vi "PiezoDAQStop.vi"(9 "error in (no error)":errorcluster) -> (0 "Last Value":dbl, 6 "error out":errorcluster)   [LabVIEW 2009]
uses:
  PiezoGlobal.vi
  Program Files/National Instruments/LabVIEW 2009/resource/objmgr/daqmx.rc
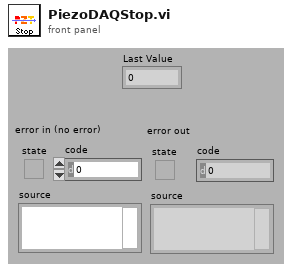
[diagram p1: front panel]
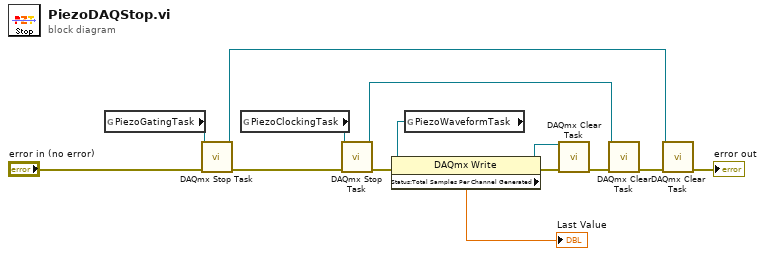
[diagram p0: block diagram]
diagram:
  n1 = global read "PiezoGlobal.vi" "PiezoGatingTask"() -> (w6:refnum<k21>)
  n2 = call <vilib>:"DAQmx Stop Task.vi"("task/channels in"=w6, "error in"="error in (no error)") -> ("task out"=w1:refnum<k21>, "error out"=w4:errorcluster)  [unwired: 12 in]
  n3 = global read "PiezoGlobal.vi" "PiezoClockingTask"() -> (w14:refnum<k21>)
  n4 = call <vilib>:"DAQmx Stop Task.vi"("task/channels in"=w14, "error in"=w4) -> ("task out"=w13:refnum<k21>, "error out"=w11:errorcluster)  [unwired: 12 in]
  n5 = global read "PiezoGlobal.vi" "PiezoWaveformTask"() -> (w10:refnum<k21>)
  n6 = property class="DAQmx Write"(reference=w10, error in=w11) -> (reference out=w9:refnum<k21>, error out=w8:errorcluster, "Status:Total Samples Per Channel Generated"=→"Last Value":dbl)
  n7 = call <vilib>:"DAQmx Clear Task.vi"("task in"=w9, "error in"=w8) -> ("error out"=w12:errorcluster)  [unwired: 13 in]
  n8 = call <vilib>:"DAQmx Clear Task.vi"("task in"=w13, "error in"=w12) -> ("error out"=w3:errorcluster)  [unwired: 13 in]
  n9 = call <vilib>:"DAQmx Clear Task.vi"("task in"=w1, "error in"=w3) -> ("error out"=→"error out":errorcluster)  [unwired: 13 in]
